vi "PC_Data Buffer.vi"(6 "Normal FGV Method":T1, 8 "error in":errorcluster, 10 "Max Size":i32, 11 "Data In":waveform(dbl)[](array[waveform])) -> (0 "error out":errorcluster, 3 "Data Out":waveform(dbl)[](array[waveform]))   [LabVIEW 2018]
uses:
  Data Def/PC_Normal FGV Method.ctl
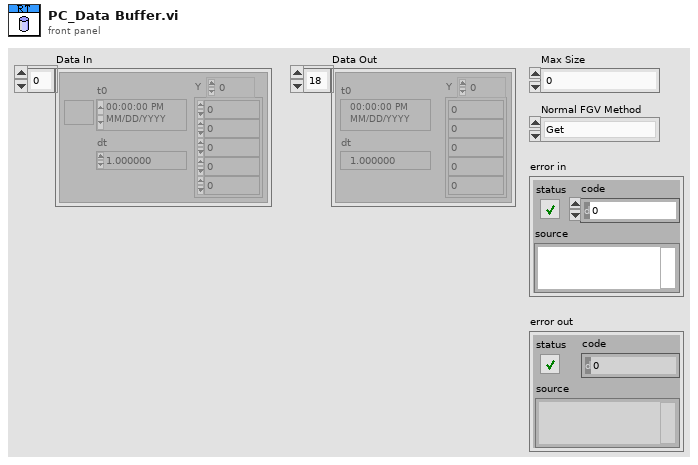
[diagram p1: front panel]
types:
  T1 = typedef "PC_Normal FGV Method.ctl" = enum16{"Get", "Put"}
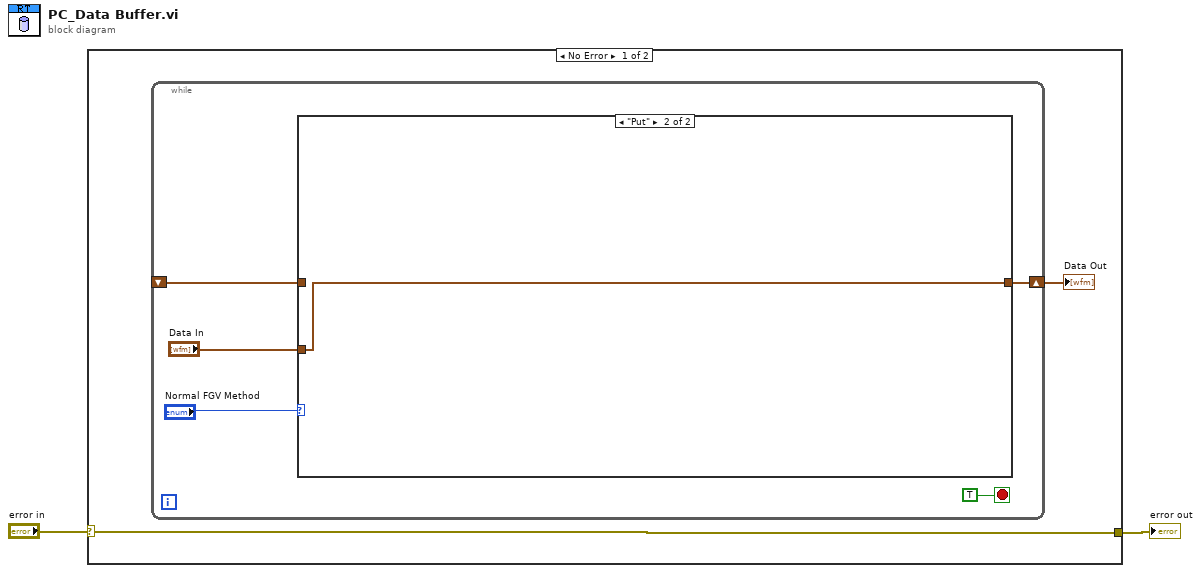
[diagram p0: block diagram]
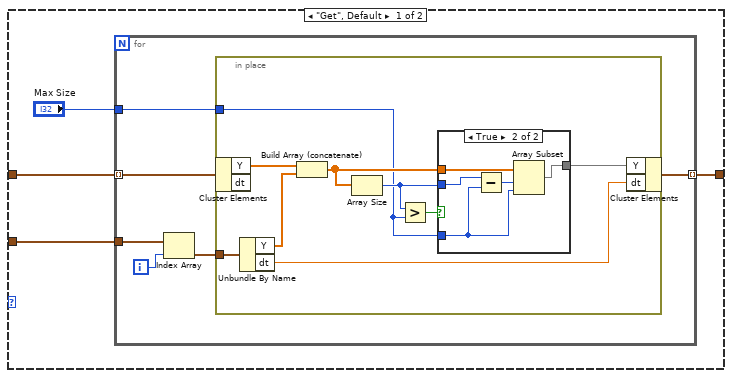
[diagram p2: hidden frame]
diagram:
  n1 = case shown="No Error" "error in" {
    selector: "error in" -> [w3 w36]
    tunnel: [w3 w36] -> w1
    frame No Error {
      n2 = while {
        shift-right: [w7] -> w4
        shift-left: _ -> [w8]
        stop <- TRUE stop-if-true
        n3 = case shown="\"Put\"" "Normal FGV Method" {
          tunnel: w8 -> [w13 _]
          tunnel: [w10 w35] -> w7
          tunnel: "Data In" -> [w11 w35]
          frame "Get", Default {
            n4 = for {
              tunnel: w11 -> [w17]
              tunnel: w13 -> [w16] mode=indexing
              tunnel: "Max Size" -> [w18]
              tunnel: [w14] -> w10 mode=indexing
              i -> [w19]
              n5 = Index Array(array=w17, index=w19) -> (element=w15:waveform(dbl))
              n6 = in-place {
                in-place-border: w18 -> [w23]
                in-place-border: w15 -> [w22]
                n7 = in-place-cluster #1(w16) -> ("Y"=w28:dbl[])  [unwired: 1 out]
                n8 = Unbundle By Name(w22) -> ("Y"=w21:dbl[], "dt"=w20:dbl)
                n9 = Build Array (concatenate)(w28, w21) -> (w25:dbl[])
                n10 = Array Size(array=w25) -> (size(s)=w27:i32)
                n11 = Greater?(x=w27, y=w23) -> (0:w26:bool)
                n12 = case shown="True" w26 {
                  tunnel: w25 -> [w29 w33]
                  tunnel: [w29 w30] -> w24
                  tunnel: w27 -> [_ w34]
                  tunnel: w23 -> [_ w31]
                  frame False {
                  }
                  frame True {
                    n13 = Subtract(x=w34, y=w31) -> (x-y=w32:i32)
                    n14 = Array Subset(array=w33, index=w32, length=w31) -> (w30:dbl[])
                  }
                }
                n15 = in-place-cluster #1("Y"=w24, "dt"=w20) -> (w14:waveform(dbl))
              }
            }
          }
          frame "Put" {
          }
        }
      }
      "Data Out" <- w4
    }
    frame Error {
    }
  }
  "error out" <- w1
